vi "Intake Controller.vi"(8 "error in":errorcluster) -> ()   [LabVIEW 2019]
doc: "This VI executes continuously carrying out the current operation and responding to updates or new operations. It will often contain the timing or control code that is difficult to place directly in TeleOp. This VI generally opens all sensors and motors and isolates the rest of the robot code from knowing how the operations are carried out."
uses:
  <vilib>/Rock Robotics/WPI/Framework/Completion Status.ctl
  Intake Setpoints.ctl
  Intake Operations.ctl
  <vilib>/Rock Robotics/WPI/Solenoid/WPI_SolenoidChannel.ctl
  <vilib>/Rock Robotics/WPI/Solenoid/WPI_SolenoidValue.ctl
  <vilib>/Rock Robotics/WPI/Solenoid/WPI_SolenoidOpenDouble.vi
  <vilib>/Rock Robotics/WPI/Solenoid/WPI_SolenoidSetEnum.vi
  <vilib>/Rock Robotics/Network Tables/NT Write Boolean.vi
panel:
  in  "Interactive Values":T1
  out "Current\nCmd":string
  in  "Buttons":cluster{"Execute Cmd":bool, "Abort Cmd":bool}
  out "Command Timing":cluster{"Start Time (ms)":u32, "Iterations":i32}
  out "Status":T3
  # "Tip: It may be helpful to observe inputs and sensor values.\nYou may also want to display tuning or debugging controls."
  # "Interactive Command: You may fill in the settings for a command\nand schedule it with the Execute button. You can observe and abort\nany command while fine tuning the code for the controller."
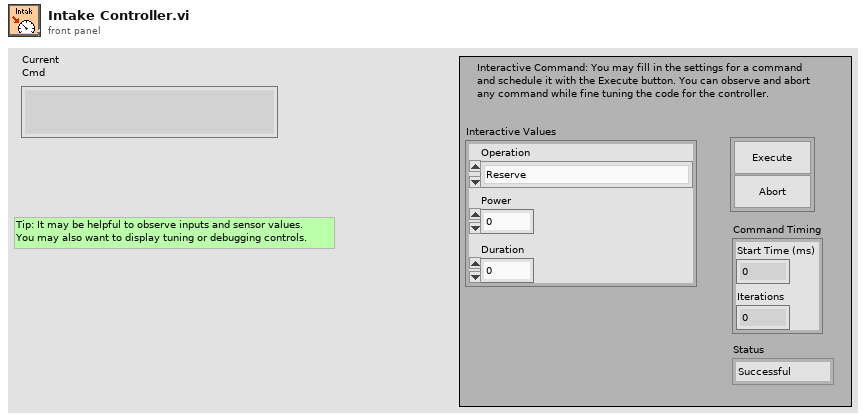
[diagram p1: front panel]
types:
  T1 = typedef "Intake Setpoints.ctl" = cluster{"Operation":T2, "Power":dbl, "Duration":dbl}
  T2 = typedef "Intake Operations.ctl" = enum16{"Reserve", "Read Current", "Immediate", "Intake for Time", "Intake Immediate", "Outtake for Time", "Outtake Immediate", "Extend Immediate", "Retract Immediate"}
  T3 = typedef "Completion Status.ctl" = enum16{"Successful", "Aborted", "Incomplete"}
  T4 = typedef "WPI_SolenoidChannel.ctl" = enum8{"Solenoid 0", "Solenoid 1", "Solenoid 2", "Solenoid 3", "Solenoid 4", "Solenoid 5", "Solenoid 6", "Solenoid 7", "Invalid"}
  T5 = typedef "WPI_MotorControlDeviceRef.ctl" = cluster{"DeviceStatus":errorcluster, "Type":T6, "PWM":cluster{"PWM Channel":T7, "DeadBand":T8}, "CAN":cluster{"Device Number":u8, "SetOutput VI Ref":variant, "GetOutput VI Ref":variant, "Enable VI Ref":variant, "Disable VI Ref":variant, "Data":variant}, "Invert":bool, "DIO PWM":cluster{"PWM \"Enable\" Channel":T7, "DIOChannel":T9, "PWM Rate":dbl}}
  T6 = typedef "WPI_MotorControlType.ctl" = enum16{"PWM", "CAN", "DIO PWM"}
  T7 = typedef "FPGA_DIOPWMChannel.ctl" = enum8{"PWM 0", "PWM 1", "PWM 2", "PWM 3", "PWM 4", "PWM 5", "PWM 6", "PWM 7", "PWM 8", "PWM 9", "PWM MXP 0", "PWM MXP 1", "PWM MXP 2", "PWM MXP 3", "PWM MXP 4", "PWM MXP 5", "PWM MXP 6", "PWM MXP 7", "PWM MXP 8", "PWM MXP 9", "Invalid"}
  T8 = typedef "WPI_PWMDeadband.ctl" = cluster{"Name":string, "maxPositivePwm":i32, "minPositivePwm":i32, "centerPwm":i32, "maxNegativePwm":i32, "minNegativePwm":i32, "angularRange":u16}
  T9 = typedef "FPGA_DIOChannel.ctl" = enum8{"DIO 0", "DIO 1", "DIO 2", "DIO 3", "DIO 4", "DIO 5", "DIO 6", "DIO 7", "DIO 8", "DIO 9", "DIO MXP 0", "DIO MXP 1", "DIO MXP 2", "DIO MXP 3", "DIO MXP 4", "DIO MXP 5", "DIO MXP 6", "DIO MXP 7", "DIO MXP 8", "DIO MXP 9", "DIO MXP 10", "DIO MXP 11", "DIO MXP 12", "DIO MXP 13", "DIO MXP 14", "DIO MXP 15", "SPI Port CS1", "SPI Port CS2", "SPI Port CS3", "SPI Port MISO", "SPI Port MOSI", "Invalid"}
  T10 = typedef "WPI_SolenoidDevRef.ctl" = cluster{"DevStatus":errorcluster, "Pneumatics Control Module":u8, "Forward Solenoid Channel":T4, "Reverse Solenoid Channel":T4}
  T11 = typedef "Command Status Info.ctl" = cluster{"Name":string, "Status":T3, "notifier out":T12}
  T12 = typedef "Completion Notifier.ctl" = refnum<notifier>
  T13 = cluster{"Current Command":T1, "Command Timing":cluster{"Start Time (ms)":u32, "Iterations":i32}, "Command Arguments":cluster{"Command Info":T11, "Description":string, "Default Command":T1, "queue out":refnum<queue>, "Subsystem Name":string}}
  T14 = typedef "WPI_SolenoidValue.ctl" = enum16{"Off", "On", "Forward", "Reverse"}
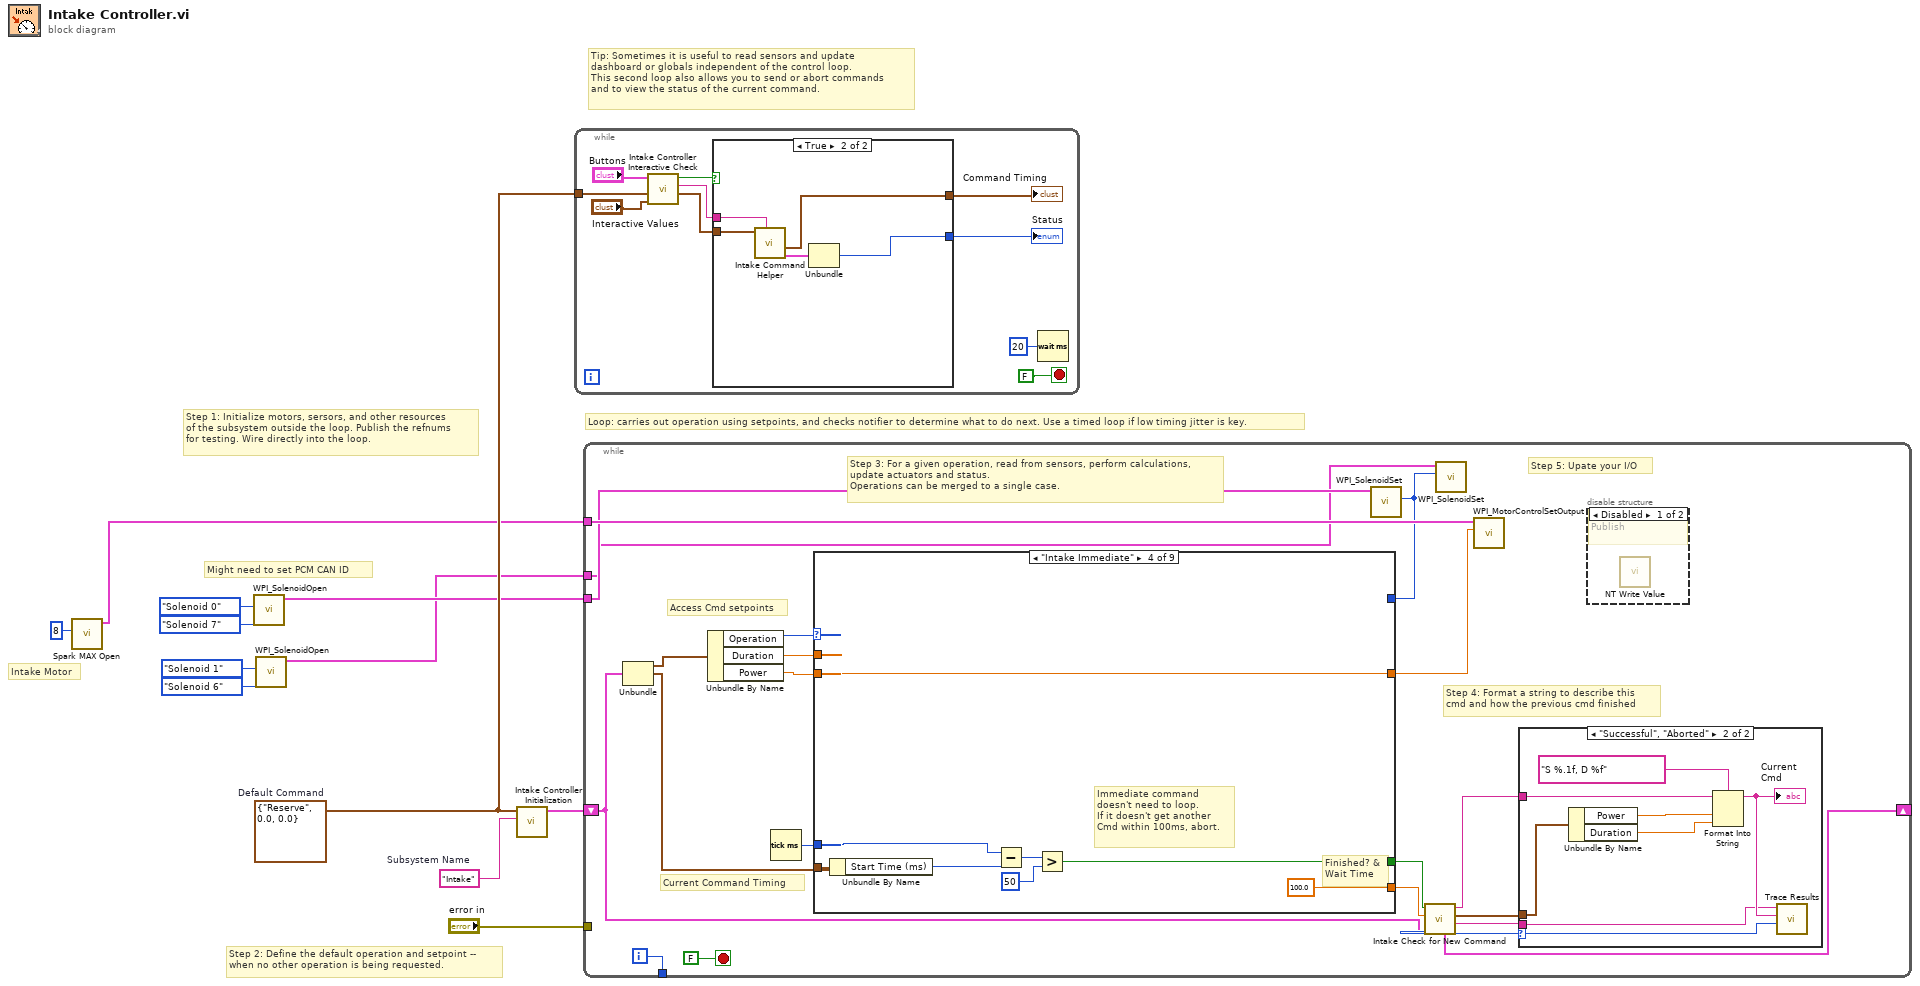
[diagram p0: block diagram]
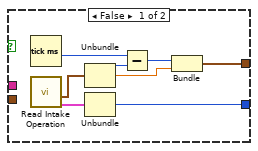
[diagram p2: hidden frame]
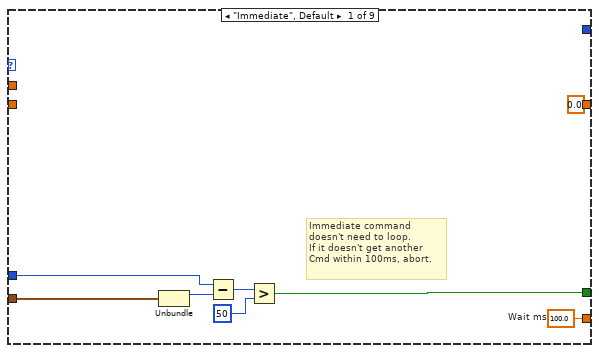
[diagram p3: hidden frame]
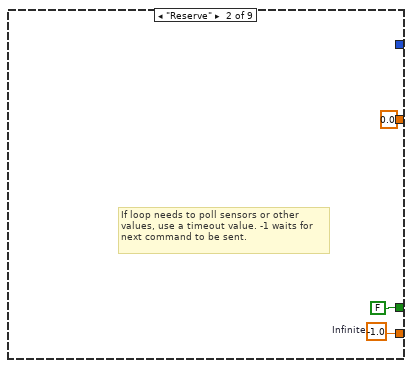
[diagram p4: hidden frame]
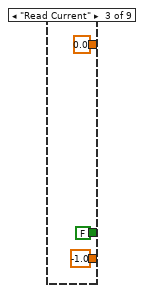
[diagram p5: hidden frame]
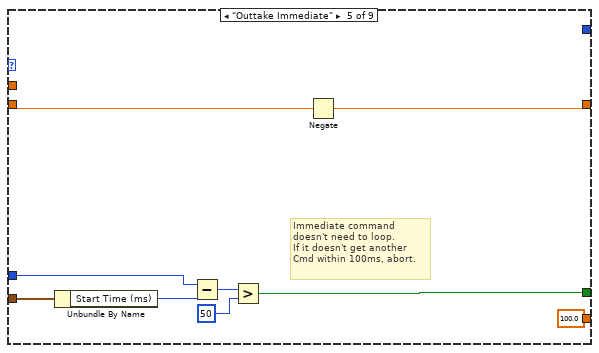
[diagram p6: hidden frame]
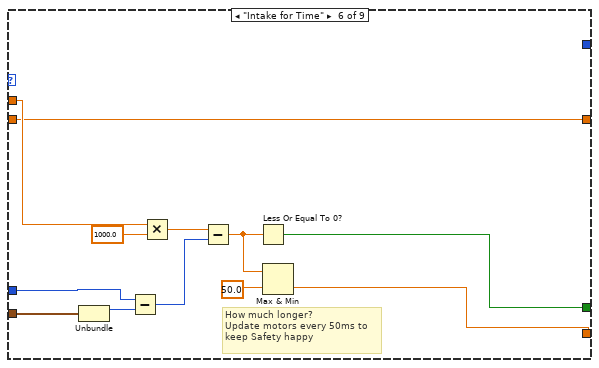
[diagram p7: hidden frame]
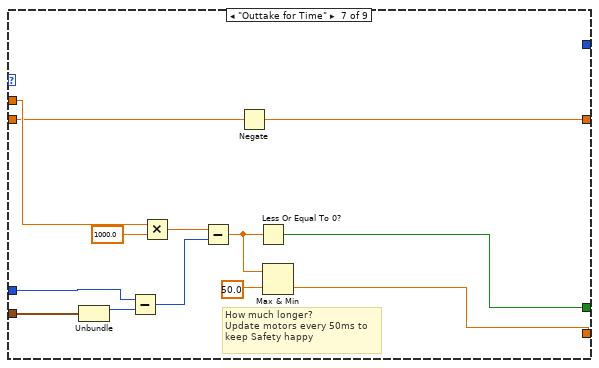
[diagram p8: hidden frame]
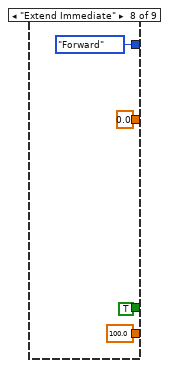
[diagram p9: hidden frame]
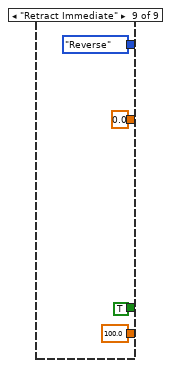
[diagram p10: hidden frame]
diagram:
  w9 = T1 {"Operation"=enum."Reserve", "Power"=0.0, "Duration"=0.0}  # Default Command
  w10 = "Intake"  # Subsystem Name
  # "Might need to set PCM CAN ID"
  # "Intake Motor"
  # "Tip: Sometimes it is useful to read sensors and update\ndashboard or globals independent of the control loop.\nThis second loop also allows you to send or abort commands\nand to view the status of the current command."
  # "Step 2: Define the default operation and setpoint --\nwhen no other operation is being requested."
  # "Step 1: Initialize motors, sersors, and other resources\nof the subsystem outside the loop. Publish the refnums\nfor testing. Wire directly into the loop."
  # "Loop: carries out operation using setpoints, and checks notifier to determine what to do next. Use a timed loop if low timing jitter is key."
  n1 = call <vilib>:"Spark MAX Open.vi"("Device Number"=u8 8) -> ("MotorControlDeviceRef"=w7:T5)  [unwired: 9 in, 1 out]
  n2 = call-poly <vilib>:"WPI_SolenoidOpen.vi"("Reverse Solenoid Channel"=WPI_SolenoidChannel."Solenoid 7", "Forward Solenoid Channel"=WPI_SolenoidChannel."Solenoid 0") -> ("SolenoidDevRef"=w2:T10)  [unwired: 8 in, 1 out]
  n3 = call-poly <vilib>:"WPI_SolenoidOpen.vi"("Reverse Solenoid Channel"=WPI_SolenoidChannel."Solenoid 6", "Forward Solenoid Channel"=WPI_SolenoidChannel."Solenoid 1") -> ("SolenoidDevRef"=w1:T10)  [unwired: 8 in, 1 out]
  n4 = call "Intake Controller Initialization.vi"("Subsystem Name"=w10, "Default Command"=w9) -> ("Current Command"=w11:T13)  [unwired: 9 in]
  n5 = while {
    tunnel: w9 -> [w19]
    stop <- FALSE stop-if-true
    n6 = call "Intake Controller Interactive Check.vi"("Interactive Command in"="Interactive Values", "Default Command"=w19, "Buttons"="Buttons") -> ("Interactive Command out"=w16:T1, "Trace String"=w17:string, "Schedule"=w18:bool)  [unwired: 6 in]
    n7 = case shown="True" w18 {
      tunnel: [w30 w35] -> w15
      tunnel: w16 -> [_ w33]
      tunnel: [w26 w31] -> w14
      tunnel: w17 -> [_ w34]
      frame False {
        n8 = Tick Count (ms)() -> (millisecond timer value=w25:u32)
        n9 = call "Read Intake Operation.vi"() -> ("Command Info"=w23:T11, "SubSystem Data"=w24:T1)  [unwired: 9 in, 1 out]
        n10 = Unbundle(w24) -> ("Operation"=w29:T2, "Power"=w27:dbl)  [unwired: 1 out]
        n11 = Unbundle(w23) -> ("Status"=w30:T3)  [unwired: 2 out]
        n12 = Subtract(x=w25, y=w29) -> (x-y=w28:u32)
        n13 = Bundle(w28, "Power"=w27) -> (w26:cluster{u32, "Power":dbl})  [unwired: 1 in]
      }
      frame True {
        n14 = call "Intake Command Helper.vi"("Description"=w34, "SubSystem Data"=w33) -> ("Command Info Out"=w32:T11, "Command Timing"=w31:cluster{"Start Time (ms)":u32, "Iterations":i32})  [unwired: 7 in, 1 out]
        n15 = Unbundle(w32) -> ("Status"=w35:T3)  [unwired: 2 out]
      }
    }
    "Status" <- w15
    "Command Timing" <- w14
    n16 = Wait (ms)(milliseconds to wait=u32 20) -> ()  [unwired: 1 out]
  }
  n17 = while {
    shift-right: [w53] -> _
    shift-left: w11 -> [w48]
    tunnel: [w55] -> _
    tunnel: "error in" -> [_]
    tunnel: w7 -> [w41]
    tunnel: w2 -> [w39]
    tunnel: w1 -> [w38]
    i -> [w55]
    stop <- FALSE stop-if-true
    # "Step 5: Upate your I/O"
    # "Step 4: Format a string to describe this\ncmd and how the previous cmd finished"
    # "Current Command Timing"
    # "Access Cmd setpoints"
    # "Finished? &\nWait Time"
    # "Step 3: For a given operation, read from sensors, perform calculations,\nupdate actuators and status.\nOperations can be merged to a single case."
    n18 = Unbundle(w48) -> ("Current Command"=w54:T1, "Command Timing"=w43:cluster{"Start Time (ms)":u32, "Iterations":i32})  [unwired: 1 out]
    n19 = Unbundle By Name(w54) -> ("Operation"=w47:T2, "Duration"=w46:dbl, "Power"=w45:dbl)
    n20 = Tick Count (ms)() -> (millisecond timer value=w44:u32)
    n21 = case shown="\"Intake Immediate\"" w47 {
      tunnel: [w64 w67 -1.0 ("Infinite") 100.0 ("Infinite") 100.0 ("Infinite") w90 w103 100.0 ("Infinite") 100.0 ("Infinite")] -> w37
      tunnel: [w58 FALSE ("ignore previous (F)") FALSE ("ignore previous (F)") w73 w82 w91 w104 TRUE ("ignore previous (F)") TRUE ("ignore previous (F)")] -> w36
      tunnel: w43 -> [w60 _ _ w71 w80 w93 w106 _ _]
      tunnel: w46 -> [_ _ _ _ _ w89 w102 _ _]
      tunnel: w44 -> [w59 _ _ w74 w81 w92 w105 _ _]
      tunnel: w45 -> [_ _ _ w78 w86 w88 w101 _ _]
      tunnel: [0.0 ("Power") 0.0 ("Power") 0.0 ("Power") w78 w87 w88 w100 0.0 ("Power") 0.0 ("Power")] -> w42
      tunnel: [_ _ _ _ _ _ _ WPI_SolenoidValue."Forward" ("Value") WPI_SolenoidValue."Reverse" ("Value")] -> w40
      frame "Immediate", Default {
        w64 = 100.0  # Wait ms
        # "Immediate command\ndoesn't need to loop.\nIf it doesn't get another\nCmd within 100ms, abort."
        n22 = Unbundle(w60) -> ("Start Time (ms)"=w63:u32)  [unwired: 1 out]
        n23 = Subtract(x=w59, y=w63) -> (x-y=w62:u32)
        n24 = Greater?(x=w62, y=u8 50 ("Left Motor")) -> (0:w58:bool)
      }
      frame "Reserve" {
        w67 = -1.0  # Infinite
        # "If loop needs to poll sensors or other\nvalues, use a timeout value. -1 waits for\nnext command to be sent."
      }
      frame "Read Current" {
      }
      frame "Intake Immediate" {
        # "Immediate command\ndoesn't need to loop.\nIf it doesn't get another\nCmd within 100ms, abort."
        n25 = Unbundle By Name(w71) -> ("Start Time (ms)"=w75:u32)
        n26 = Subtract(x=w74, y=w75) -> (x-y=w77:u32)
        n27 = Greater?(x=w77, y=u8 50 ("Left Motor")) -> (0:w73:bool)
      }
      frame "Outtake Immediate" {
        # "Immediate command\ndoesn't need to loop.\nIf it doesn't get another\nCmd within 100ms, abort."
        n28 = Unbundle By Name(w80) -> ("Start Time (ms)"=w79:u32)
        n29 = Subtract(x=w81, y=w79) -> (x-y=w84:u32)
        n30 = Greater?(x=w84, y=u8 50 ("Left Motor")) -> (0:w82:bool)
        n31 = Negate(x=w86) -> (-x=w87:dbl)
      }
      frame "Intake for Time" {
        # "How much longer?\nUpdate motors every 50ms to\nkeep Safety happy"
        n32 = Unbundle(w93) -> ("Start Time (ms)"=w96:u32)  [unwired: 1 out]
        n33 = Subtract(x=w92, y=w96) -> (x-y=w99:u32)
        n34 = Multiply(x=w89, y=1000.0) -> (x*y=w98:dbl)
        n35 = Subtract(x=w98, y=w99) -> (x-y=w95:dbl)
        n36 = Less Or Equal To 0?(x=w95) -> (x <= 0?=w91:bool)
        n37 = Max & Min(x=w95, y=50.0) -> (min(x,y)=w90:dbl)  [unwired: 1 out]
      }
      frame "Outtake for Time" {
        # "How much longer?\nUpdate motors every 50ms to\nkeep Safety happy"
        n38 = Unbundle(w106) -> ("Start Time (ms)"=w109:u32)  [unwired: 1 out]
        n39 = Subtract(x=w105, y=w109) -> (x-y=w112:u32)
        n40 = Multiply(x=w102, y=1000.0) -> (x*y=w111:dbl)
        n41 = Subtract(x=w111, y=w112) -> (x-y=w108:dbl)
        n42 = Negate(x=w101) -> (-x=w100:dbl)
        n43 = Less Or Equal To 0?(x=w108) -> (x <= 0?=w104:bool)
        n44 = Max & Min(x=w108, y=50.0) -> (min(x,y)=w103:dbl)  [unwired: 1 out]
      }
      frame "Extend Immediate" {
      }
      frame "Retract Immediate" {
      }
    }
    n45 = call-poly <vilib>:"WPI_SolenoidSet.vi"("Value"=w40, "SolenoidDevRef"=w39) -> ()  [unwired: 8 in, 2 out]
    n46 = call "Intake Check for New Command.vi"("Current Command"=w48, "Wait time (ms)"=w37, "Finished?"=w36) -> ("Completion"=w49:T3, "Subsystem Name"=w50:string, "Current Command"=w51:T1, "Initial Trace String"=w52:string, "NextCommand"=w53:T13)  [unwired: 4 in]
    n47 = call-poly <vilib>:"WPI_SolenoidSet.vi"("Value"=w40, "SolenoidDevRef"=w38) -> ()  [unwired: 8 in, 2 out]
    n48 = call <vilib>:"WPI_MotorControlSetOutput.vi"("Output"=w42, "MotorControlDevRef"=w41) -> ()  [unwired: 7 in, 3 out]
    n49 = case shown="\"Successful\", \"Aborted\"" w49 {
      selector: w49 -> [_ w128]
      tunnel: w52 -> [_ w124]
      tunnel: w51 -> [_ w125]
      tunnel: w50 -> [_ w121]
      frame "Incomplete", Default {
        # "Continuing current command"
      }
      frame "Successful", "Aborted" {
        # "Report and setup for next command"
        n50 = Unbundle By Name(w125) -> ("Power"=w127:dbl, "Duration"=w122:dbl)
        n51 = Format Into String(format string="S %.1f, D %f", initial string=w124, w127, w122) -> (resulting string=w123:string)  [unwired: 1 in, 1 out]
        "Current\nCmd" <- w123
        n52 = call <vilib>:"Trace Results.vi"("Status of previous command"=w128, "Description"=w123, "Subsystem"=w121) -> ()  [unwired: 9 in]
      }
    }
    n53 = disable-structure shown="Disabled" {
      frame Disabled {
        # "Publish"
        n54 = call-poly <vilib>:"NT Write Value.vi"() -> ()  [unwired: 11 in, 1 out]
      }
      frame Enabled {
      }
    }
  }
